vi "lineFilter.vi"(9 "min line size":i32, 10 "Input":cluster{"Line":cluster{"X":dbl, "Y":dbl}[]}[](array[cluster])) -> (2 "Output":cluster{"Line":cluster{"X":dbl, "Y":dbl}[]}[](array[cluster]))   [LabVIEW 2016]
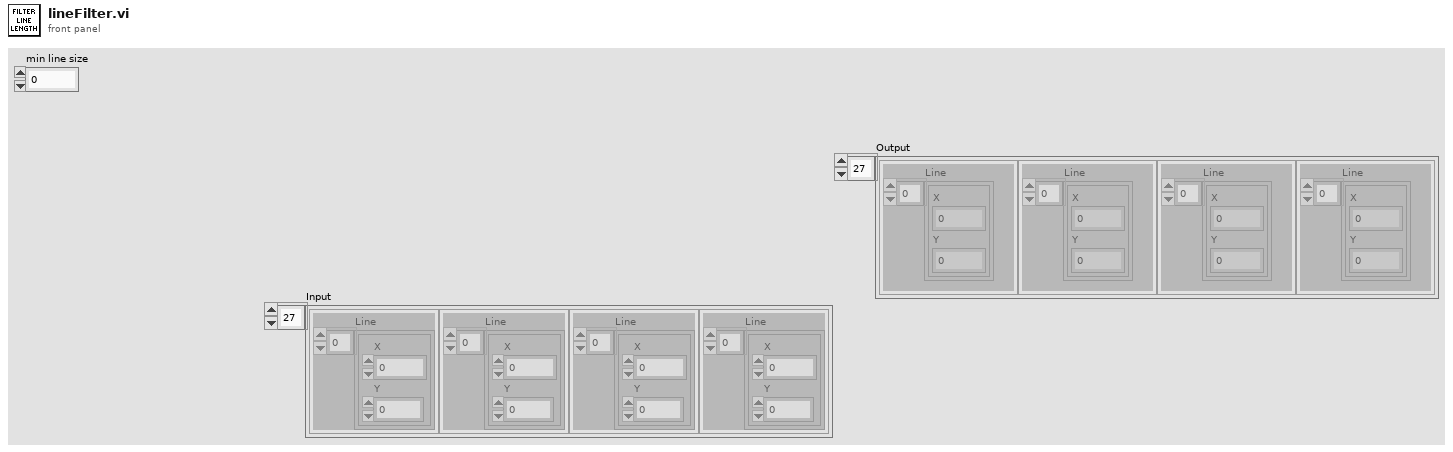
[diagram p1: front panel]
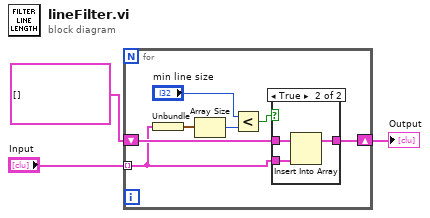
[diagram p0: block diagram]
diagram:
  n1 = for {
    shift-right: [w5] -> w1
    shift-left: cluster{"Line":cluster{"X":dbl, "Y":dbl}[]}[] [] -> [w6]
    tunnel: "Input" -> [w4] mode=indexing
    n2 = Unbundle(w4) -> ("Line"=w10:cluster{"X":dbl, "Y":dbl}[])
    n3 = Array Size(array=w10) -> (size(s)=w9:i32)
    n4 = Less?(x="min line size", y=w9) -> (x < y?=w7:bool)
    n5 = case shown="True" w7 {
      tunnel: w6 -> [w11 w14]
      tunnel: [w11 w13] -> w5
      tunnel: w4 -> [_ w12]
      frame False {
      }
      frame True {
        n6 = Insert Into Array(array=w14, new element=w12) -> (w13:cluster{"Line":cluster{"X":dbl, "Y":dbl}[]}[])  [unwired: 1 in]
      }
    }
  }
  "Output" <- w1
